vi "ATECC2 System Designer.vi"() -> ()   [LabVIEW 2023]
uses:
  Option Type Defs/Full System Configuration.ctl
  Option Type Defs/Rack.ctl
  Option Type Defs/Middle Rail.ctl
  Option Type Defs/Ballast.ctl
  Option Type Defs/Rear Panel IO.ctl
  Option Type Defs/Panel IO Configuration.ctl
  Option Type Defs/Parts List.ctl
  <vilib>/ErrorRing/Error Ring.xnode
  <userlib>/_OpenG.lib/lvdata/lvdata.llb/openg_variant.lvlib
panel:
  out "Parts List":T1[](array[typedef])
  out "Current Configuration":T2 {"Ballast"."Side" max=5 step=1; "Ballast"."Small" max=5 step=1; "Ballast"."Main" max=5 step=1}
  in  "Full System Configuration":T2 {"Ballast"."Side" max=5 step=1; "Ballast"."Small" max=5 step=1; "Ballast"."Main" max=5 step=1}
  # "Rear panel I/O: Select one of the three major part numbers (fully, partial, blank).\nIf yoiu want custom, select the far right main panel and chose your piece-meal parts from the table below the Rear I/O secion."
  # "Front panel I/O just needs individual part numbers for I/O sub panels."
  # "1 DC 600 per AC PDU in system\n1 DC1200 per AC PDU in system"
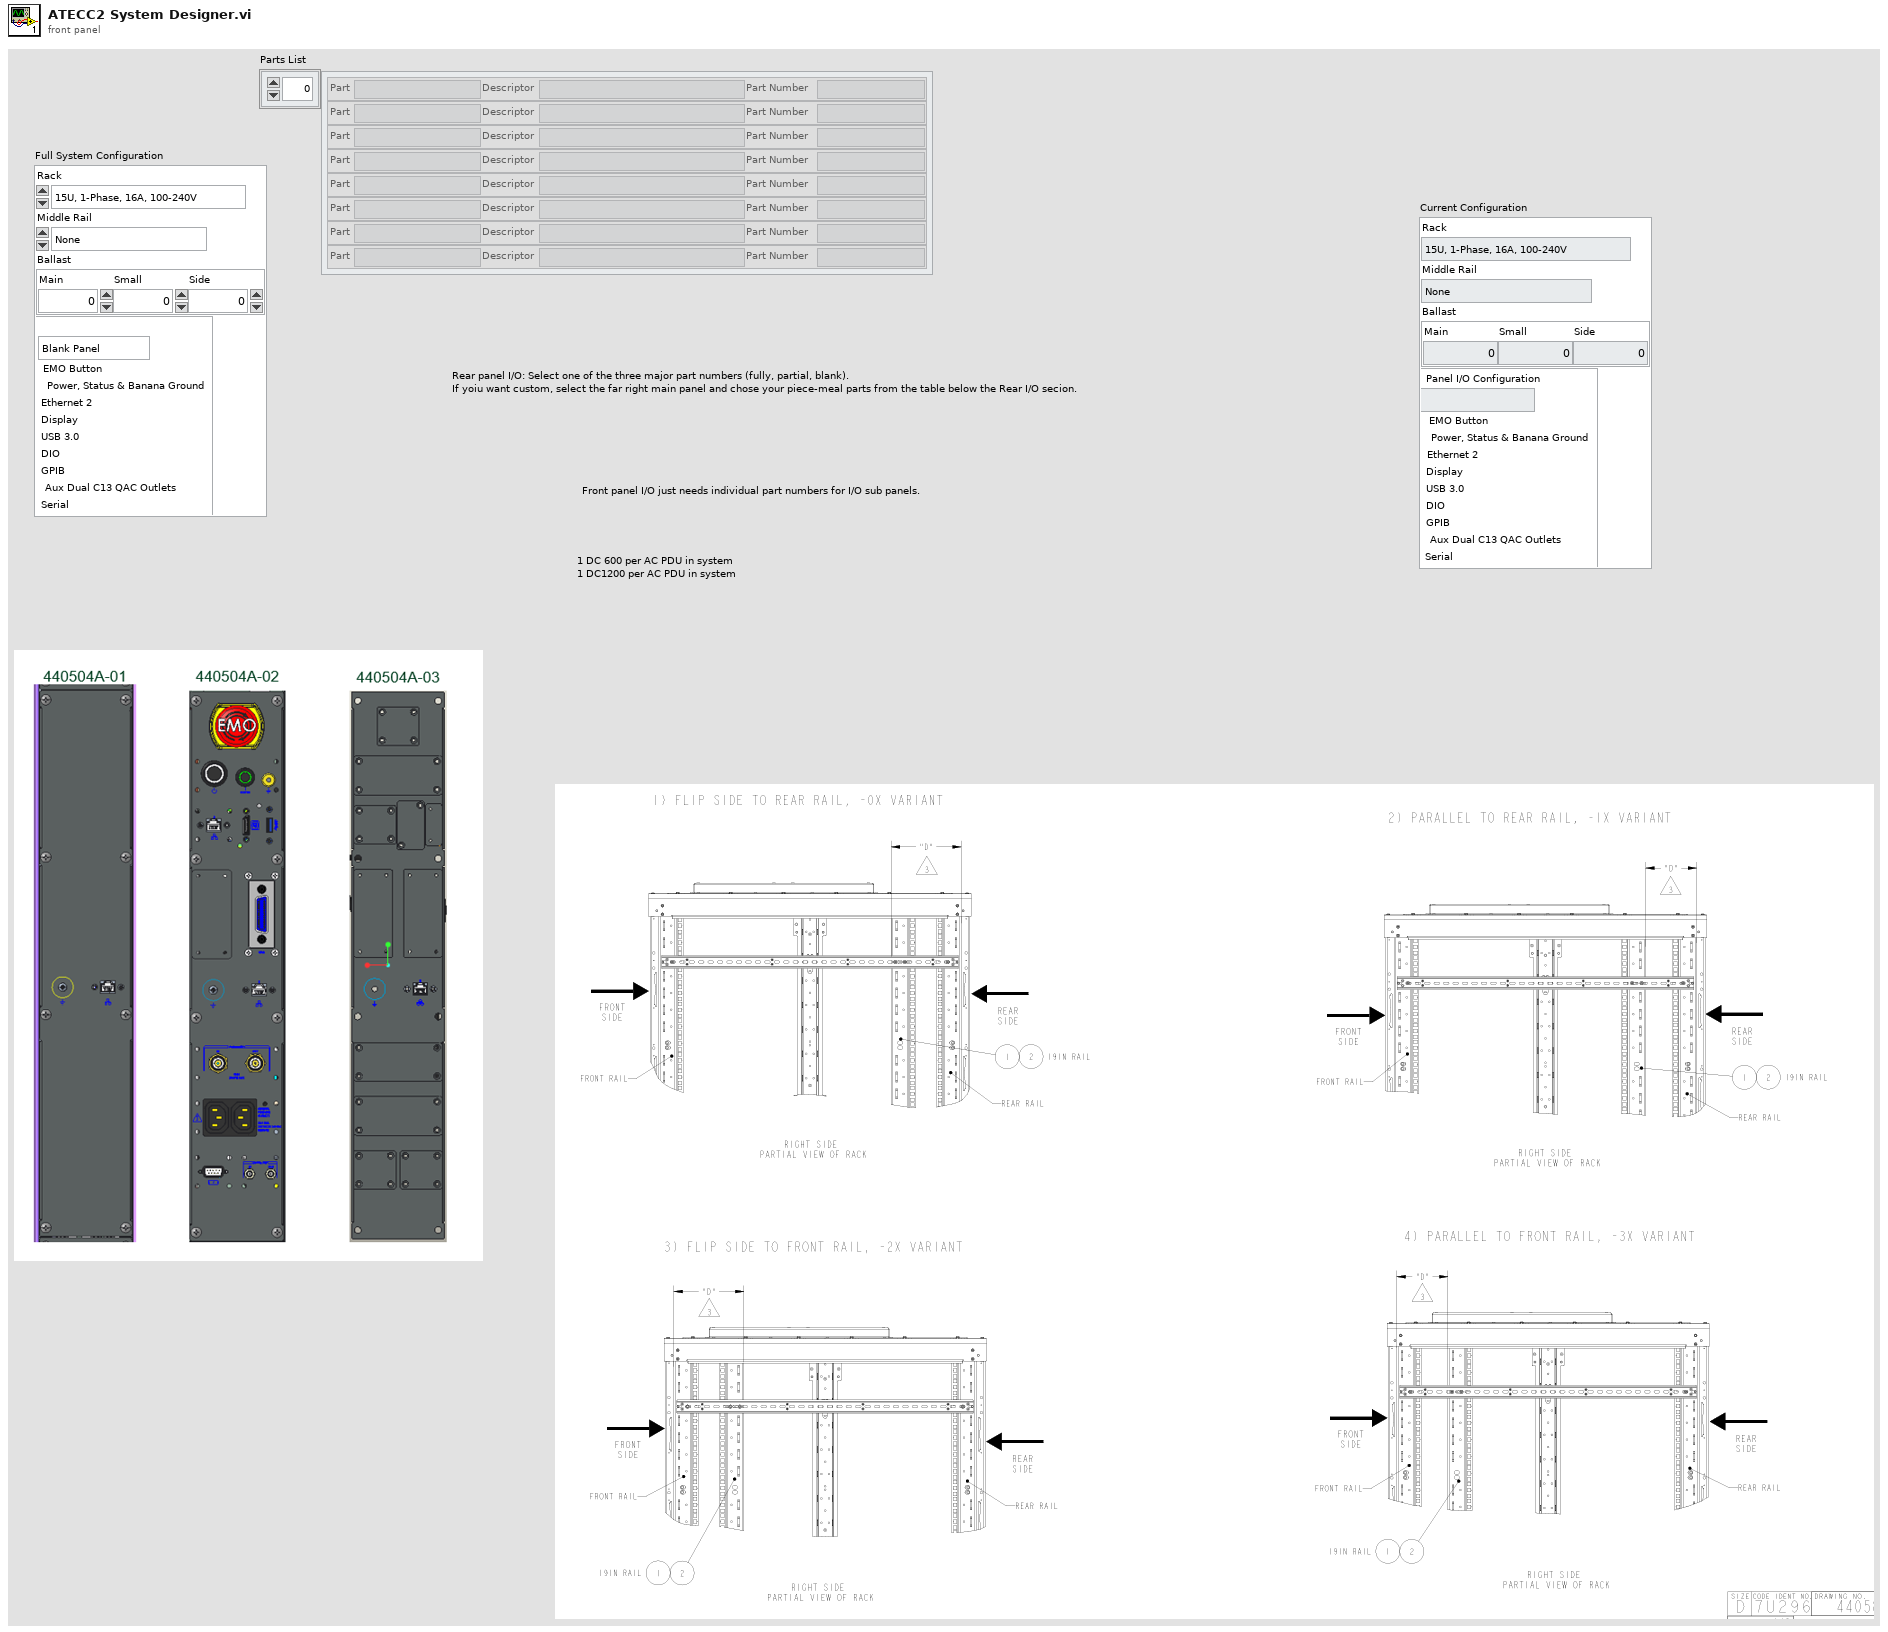
[diagram p1: front panel]
types:
  T1 = typedef "Parts List.ctl" = cluster{"Part":string, "Descriptor":string, "Part Number":string}
  T2 = typedef "Full System Configuration.ctl" = cluster{"Rack":T3, "Middle Rail":T4, "Ballast":T5, "Rear Panel I/O":T6}
  T3 = typedef "Rack.ctl" = enum16{"15U, 1-Phase, 16A, 100-240V", "15U, 1-Phase, 24A, 100-240V", "38U, 3-Phase Delta, 50A, 200-240V", "38U, 1-Phase, 24A, 100-120V", "38U, 3-Phase Wye, 50A, 200-240V", "38U, 3-Phase Delta, 50A, 380-480V", "38U, 3-Phase Delta, 32A, 200-240V", "38U, 3-Phase Wye, 16A, 100-240V", "44U, 1-Phase, 24A, 100-240V", "44U, 3-Phase Delta, 32A, 200-240V"}
  T4 = typedef "Middle Rail.ctl" = enum16{"None", "Flip Side Rear, D=168.83mm", "Parallel Rear, D=145mm", "Flip Side Front, D=145mm", "Parallel Front, D=145mm"}
  T5 = typedef "Ballast.ctl" = cluster{"Main":u16, "Small":u16, "Side":u16}
  T6 = typedef "Rear Panel IO.ctl" = cluster{"Panel I/O Configuration":T7, "Ethernet 3":bool, "Ethernet 4":bool, "Ethernet 2":bool, "Display":bool, "USB 3.0":bool, "DIO":bool, "GPIB":bool, "Aux Dual C13 QAC Outlets":bool, "Serial":bool, "SMA":bool}
  T7 = typedef "Panel IO Configuration.ctl" = enum16{"Blank Panel", "Fully Populated Panel", "Custom Panel"}
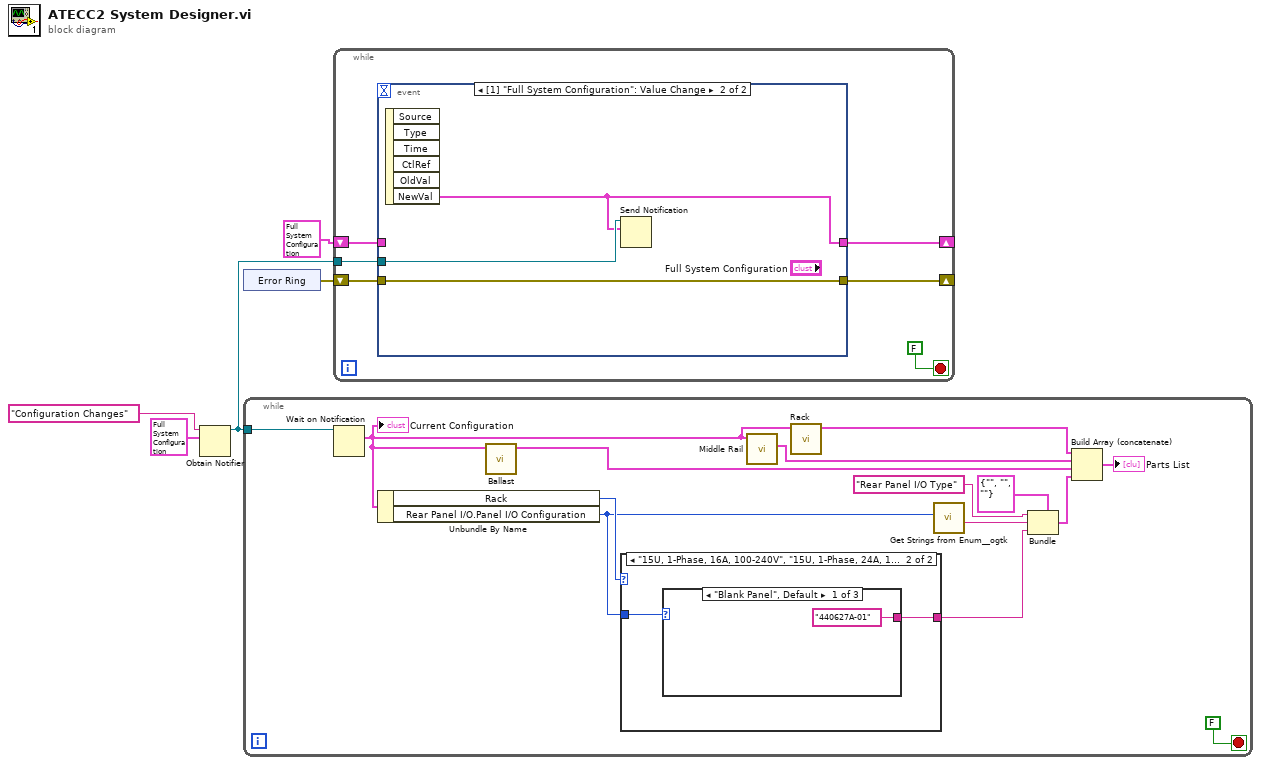
[diagram p0: block diagram]
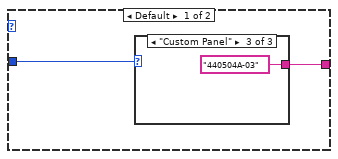
[diagram p2: hidden frame]
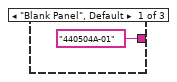
[diagram p3: hidden frame]
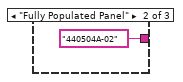
[diagram p4: hidden frame]
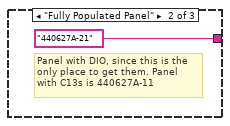
[diagram p5: hidden frame]
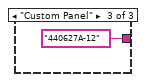
[diagram p6: hidden frame]
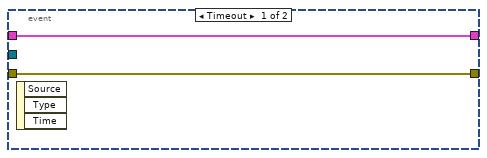
[diagram p7: hidden frame]
diagram:
  n1 = Obtain Notifier(name (unnamed)="Configuration Changes", notification data type=T2 {"Rack"=enum."15U, 1-Phase, 16A, 100-240V", "Middle Rail"=enum."None", "Ballast"={"Main"=0, "Small"=0, "Side"=0}, "Rear Panel I/O"={"Panel I/O Configuration"=enum."Blank Panel", "Ethernet 3"=FALSE, "Ethernet 4"=FALSE, "Ethernet 2"=FALSE, "Display"=FALSE, "USB 3.0"=FALSE, "DIO"=FALSE, "GPIB"=FALSE, "Aux Dual C13 QAC Outlets"=FALSE, "Serial"=FALSE, "SMA"=FALSE}} ("Full System Configuration")) -> (notifier out=w2:refnum<notifier>)  [unwired: 2 in, 2 out]
  n2 = xnode "Error Ring"() -> ("error out"=w5:errorcluster)
  n3 = while {
    tunnel: w2 -> [w19]
    stop <- FALSE stop-if-true
    n4 = Wait on Notification(notifier=w19) -> (notification=w13:T2)  [unwired: 3 in, 3 out]
    "Current Configuration" <- w13
    n5 = Unbundle By Name(w13) -> ("Rack"=w12:T3, "Rear Panel I/O.Panel I/O Configuration"=w9:T7)
    n6 = call "Ballast.vi"("Full System Configuration"=w13) -> ("Array"=w14:T1[])  [unwired: 10 in]
    n7 = case shown="\"15U, 1-Phase, 16A, 100-240V\", \"15U, 1-Phase, 24A, 100-240V\"" w12 {
      tunnel: w9 -> [w21 w26]
      tunnel: [w20 w25] -> w7
      frame Default {
        n8 = case shown="\"Custom Panel\"" w21 {
          tunnel: ["440504A-01" "440504A-02" "440504A-03"] -> w20
          frame "Blank Panel", Default {
          }
          frame "Fully Populated Panel" {
          }
          frame "Custom Panel" {
          }
        }
      }
      frame "15U, 1-Phase, 16A, 100-240V", "15U, 1-Phase, 24A, 100-240V" {
        n9 = case shown="\"Blank Panel\", Default" w26 {
          tunnel: ["440627A-01" "440627A-21" "440627A-12"] -> w25
          frame "Blank Panel", Default {
          }
          frame "Fully Populated Panel" {
            # "Panel with DIO, since this is the only place to get them. Panel with C13s is 440627A-11"
          }
          frame "Custom Panel" {
          }
        }
      }
    }
    n10 = call "Middle Rail.vi"("Full System Configuration"=w13) -> ("cluster"=w15:T1)  [unwired: 10 in]
    n11 = call "Rack.vi"("Full System Configuration"=w13) -> ("cluster"=w17:T1)  [unwired: 10 in]
    n12 = call <userlib>:"Get Strings from Enum__ogtk.vi"("Enum"=w9) -> ("String Value"=w8:string)  [unwired: 7 in, 3 out]
    n13 = Bundle(cluster=T1 {"Part"="", "Descriptor"="", "Part Number"=""}, "Part"="Rear Panel I/O Type", "Descriptor"=w8, "Part Number"=w7) -> (w6:T1)
    n14 = Build Array (concatenate)(w17, w15, w14, w6) -> (→"Parts List":T1[])
  }
  n15 = while {
    shift-right: [w35] -> _
    shift-left: w5 -> [w34]
    shift-right: [w33] -> _
    shift-left: T2 {"Rack"=enum."15U, 1-Phase, 16A, 100-240V", "Middle Rail"=enum."None", "Ballast"={"Main"=0, "Small"=0, "Side"=0}, "Rear Panel I/O"={"Panel I/O Configuration"=enum."Blank Panel", "Ethernet 3"=FALSE, "Ethernet 4"=FALSE, "Ethernet 2"=FALSE, "Display"=FALSE, "USB 3.0"=FALSE, "DIO"=FALSE, "GPIB"=FALSE, "Aux Dual C13 QAC Outlets"=FALSE, "Serial"=FALSE, "SMA"=FALSE}} ("Full System Configuration") -> [w32]
    tunnel: w2 -> [w30]
    stop <- FALSE stop-if-true
    n16 = event shown="[1] \"Full System Configuration\": Value Change" {
      selector: _ -> [_ _]
      dyn-events: _ -> [_ _]
      timeout: _ -> [_ _]
      tunnel: [w37 w40] -> w35
      tunnel: w34 -> [w37 w40]
      tunnel: [w36 w38] -> w33
      tunnel: w32 -> [w36 _]
      tunnel: w30 -> [_ w39]
      event Timeout {
        n17 = event-data() -> ()  [unwired: 1 in, 3 out]
      }
      event Value Change {
        n18 = event-data() -> ("NewVal"=w38:T2)  [unwired: 1 in, 5 out]
        n19 = Send Notification(notification=w38, notifier=w39) -> ()  [unwired: 1 in, 2 out]
      }
    }
  }
